vi "反控仪器参数公式.vi"(8 "错误输入（无错误）":errorcluster, 10 "公式":cluster{"X^2":dbl, "X":dbl, "b":dbl}, 11 "参数":string) -> (0 "错误输出":errorcluster, 3 "超时？":bool)   [LabVIEW 2016, in "MB SLAVE.lvlib"]
uses:
  MB SLAVE.lvlib
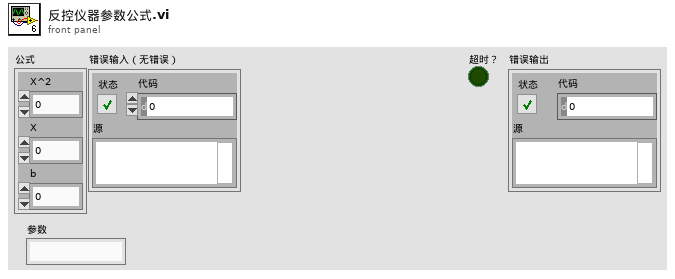
[diagram p1: front panel]
types:
  T1 = cluster{"chose":string, "公式":cluster{"X^2":dbl, "X":dbl, "b":dbl}}
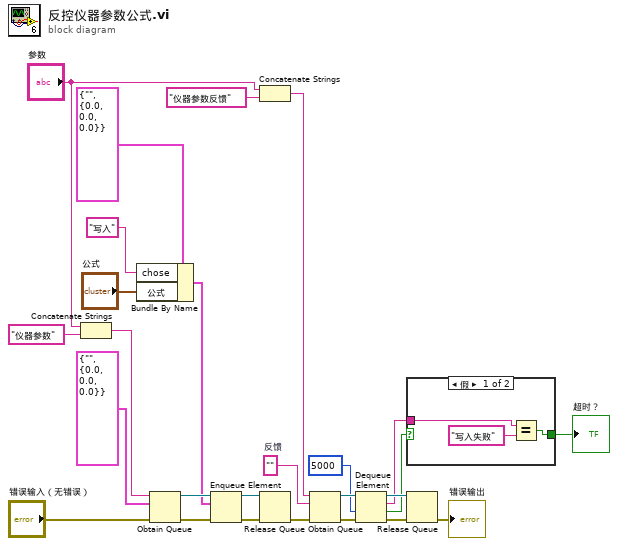
[diagram p0: block diagram]
diagram:
  w26 = ""  # 反馈
  n1 = Concatenate Strings("参数", "仪器参数" ("名称（未命名）")) -> (w1:string)
  n2 = Bundle By Name(cluster=T1 {"chose"="", "公式"={"X^2"=0.0, "X"=0.0, "b"=0.0}}, "chose"="写入", "公式"="公式") -> (w20:T1)
  n3 = Obtain Queue(name (unnamed)=w1, element data type=T1 {"chose"="", "公式"={"X^2"=0.0, "X"=0.0, "b"=0.0}}, error in (no error)="错误输入（无错误）") -> (queue out=w25:refnum<queue>, error out=w24:errorcluster)  [unwired: 2 in, 1 out]
  n4 = Enqueue Element(queue=w25, element=w20, error in (no error)=w24) -> (queue out=w18:refnum<queue>, error out=w17:errorcluster)  [unwired: 1 in, 1 out]
  n5 = Concatenate Strings("参数", "仪器参数反馈" ("名称（未命名）")) -> (w2:string)
  n6 = Release Queue(queue=w18, error in (no error)=w17) -> (error out=w16:errorcluster)  [unwired: 1 in, 2 out]
  n7 = Obtain Queue(name (unnamed)=w2, element data type=w26, error in (no error)=w16) -> (queue out=w15:refnum<queue>, error out=w14:errorcluster)  [unwired: 2 in, 1 out]
  n8 = Dequeue Element(queue=w15, timeout in ms (-1)=5000 ("超时毫秒(-1)"), error in (no error)=w14) -> (queue out=w11:refnum<queue>, element=w10:string, timed out?=w9:bool, error out=w12:errorcluster)
  n9 = case shown="假" w9 {
    selector: w9 -> [_ w30]
    tunnel: w10 -> [w28 _]
    tunnel: [w27 w30] -> w8
    frame False {
      n10 = Equal?(x=w28, y="写入失败") -> (x = y?=w27:bool)
    }
    frame True {
    }
  }
  "超时？" <- w8
  n11 = Release Queue(queue=w11, error in (no error)=w12) -> (error out=→"错误输出":errorcluster)  [unwired: 1 in, 2 out]
